vi "Actor Core.vi"(8 "error in":errorcluster, 11 "Network Stream Writer in":refnum<class "Network Stream Writer.lvclass">) -> (0 "error out":errorcluster, 3 "Actor out":refnum<class "Actor.lvclass">)   [LabVIEW 2014, in "Network Stream Writer.lvlib" / "Network Stream Writer.lvclass"]
doc: "(<B>Filename</B>: Actor Framework.lvlib:Actor.lvclass:Actor Core.vi)\n\nReceives messages to the actor, reacts to them, and initiates any error handling that may shut the actor down.\n\nDescendant classes may override this VI to append parallel tasks for the actor to complete while it handles messages. Overrides use the Call Parent Method node."
uses:
  Network Stream Writer.lvclass
  <vilib>/ActorFramework/Actor/Actor.lvclass
  Network Stream Writer Messages/Check Endpoint Msg/Check Endpoint Msg.lvclass
  <vilib>/ActorFramework/Actor/Actor.lvclass/Actor.ctl
  <vilib>/ActorFramework/Message Enqueuer/Message Enqueuer.lvclass/Message Enqueuer.ctl
  <vilib>/ActorFramework/Time-Delayed Send Message/Time-Delay Override Options.ctl
  <vilib>/ActorFramework/Message Enqueuer/Init from Existing Queue.vi
  Network Stream/Network Stream/Network Stream.lvclass
  <vilib>/ActorFramework/Message Enqueuer/Message Enqueuer.lvclass
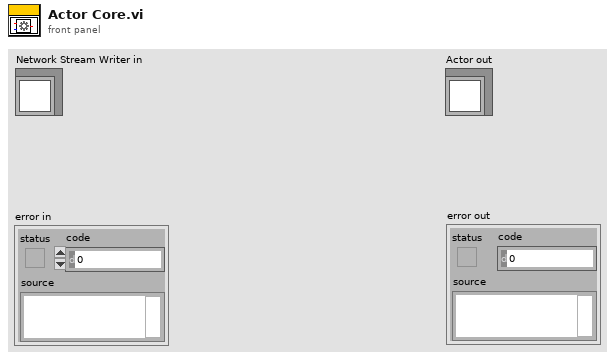
[diagram p1: front panel]
types:
  T1 = typedef "Time-Delay Override Options.ctl" = enum16{"Send next copy now", "Skip next scheduled copy", "Send next copy now and stop all further copies", "Stop all further copies"}
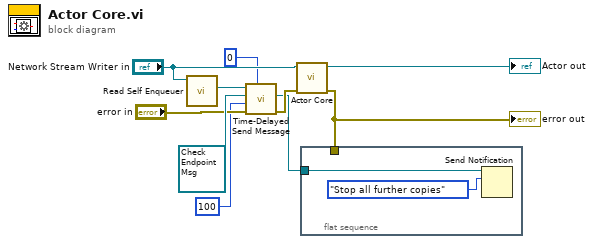
[diagram p0: block diagram]
diagram:
  n1 = call <vilib>:"Read Self Enqueuer.vi"("Actor"="Network Stream Writer in") -> ("Self Enqueuer"=w5:refnum<class "Message Enqueuer.lvclass">)  [unwired: 10 in]
  n2 = call <vilib>:"Time-Delayed Send Message.vi"("# Copies (0 = infinite repeat)"=u32 0, "error in (no error)"="error in", "Milliseconds To Wait"=100, "Message"=refnum<class "Check Endpoint Msg.lvclass"> refnum ("Network Stream Writer.lvlib:Check Endpoint Msg.lvclass"), "Message Enqueuer"=w5) -> ("error out"=w6:errorcluster, "Delivery Notifier"=w3:refnum<notifier>)  [unwired: 5 in]
  n3 = call-parent "Actor Core.vi"("error in"=w6, "Actor in"="Network Stream Writer in") -> ("error out"=w2:errorcluster, "Actor out"=→"Actor out":refnum<class "Actor.lvclass">)  [unwired: 8 in]
  "error out" <- w2
  n4 = flat-sequence {
    tunnel: w3 -> [w12]
    tunnel: w2 -> [_]
    frame #0 {
      n5 = Send Notification(notification=Time-Delay_Override_Options."Stop all further copies", notifier=w12) -> ()  [unwired: 1 in, 2 out]
    }
  }
